vi "Write Keithley user configuration.vi"(8 "error in (no error)":errorcluster, 10 "Keithley user configurations":T1={"Range (-1: auto)"=2.0, "Integration Time (NPLCs)"=1.0, "Function"=enum."VOLTAGE", "W Offset comp"=FALSE, "4-wire W"=FALSE, "Scale"=1.0, "Offset"=0.0} {"Integration Time (NPLCs)" min=0.01 max=10.0 step=0.01 format="%.2f"}, 11 "Keithley Driver in":refnum<class "Keithley Driver.lvclass">) -> (0 "error out":errorcluster, 3 "Keithley Driver out":refnum<class "Keithley Driver.lvclass">)   [LabVIEW 2016, in "Keithley Driver.lvclass"]
uses:
  Keithley Driver.lvclass
  C:/github/NHMFL_Core/Libraries/Instruments/Instrument Driver/Instrument Driver.lvclass
  Meter/Keithley Meter Parameters.ctl
  Meter/KeithleyMeter Function.ctl
  Instrument Driver/Write User configuration.vi
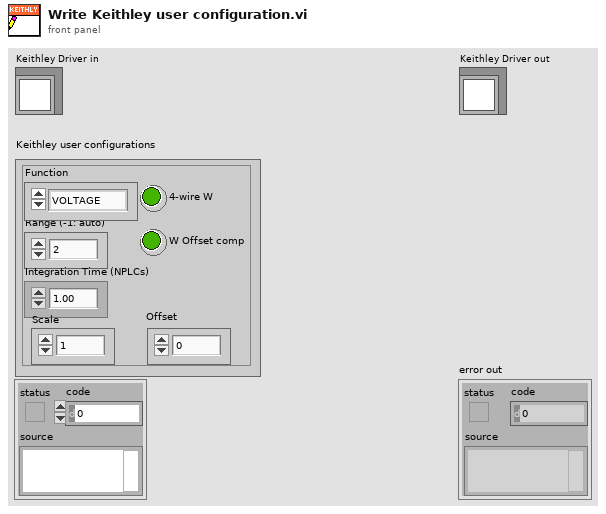
[diagram p1: front panel]
types:
  T1 = typedef "Keithley Meter Parameters.ctl" = cluster{"Range (-1: auto)":dbl, "Integration Time (NPLCs)":dbl, "Function":T2, "W Offset comp":bool, "4-wire W":bool, "Scale":dbl, "Offset":dbl}
  T2 = typedef "KeithleyMeter Function.ctl" = enum16{"VOLTAGE", "CURRENT", "RESISTANCE"}
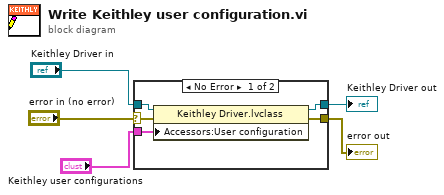
[diagram p0: block diagram]
diagram:
  n1 = case shown="No Error" "error in (no error)" {
    selector: "error in (no error)" -> [w8 w11]
    tunnel: [w7 w11] -> w4
    tunnel: [w6 w12] -> w2
    tunnel: "Keithley Driver in" -> [w10 w12]
    tunnel: "Keithley user configurations" -> [w9 _]
    frame No Error {
      n2 = property class="Keithley Driver.lvclass"(reference=w10, error in=w8, "Accessors:User configuration"=w9) -> (reference out=w6:refnum<class "Keithley Driver.lvclass">, error out=w7:errorcluster)
    }
    frame Error {
    }
  }
  "error out" <- w4
  "Keithley Driver out" <- w2
